vi "界面设计_灯.vi"(11 "停止":bool) -> (0 "布尔":bool, 1 "布尔 2":bool, 2 "布尔 4":bool, 3 "布尔 3":bool, 6 "布尔 5":bool, 8 "布尔 6":bool, 10 "布尔 8":bool, 12 "布尔 7":bool, 14 "布尔 9":bool, 15 "布尔 10":bool, 16 "布尔 12":bool, 17 "布尔 11":bool)   [LabVIEW 2019]
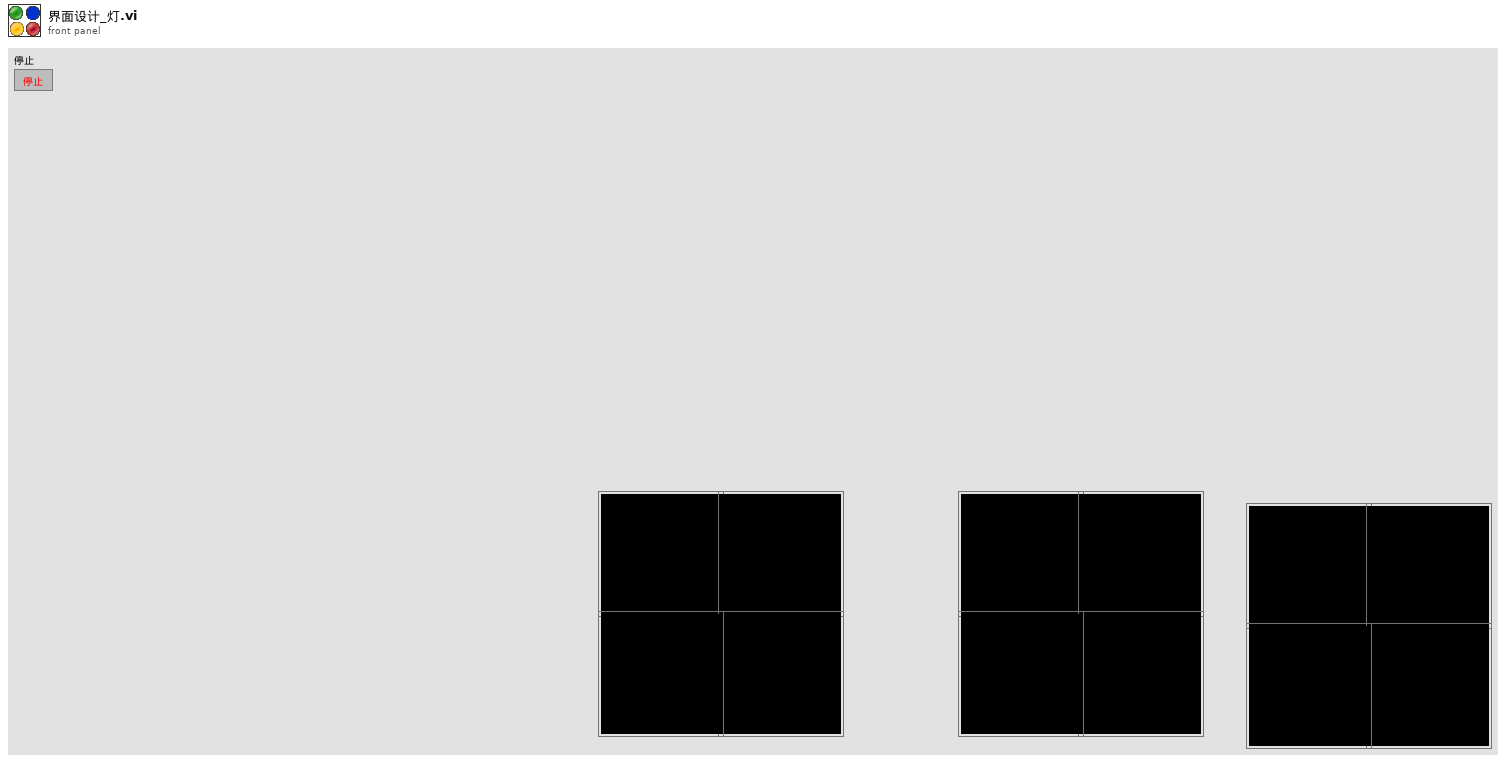
[diagram p1: front panel]
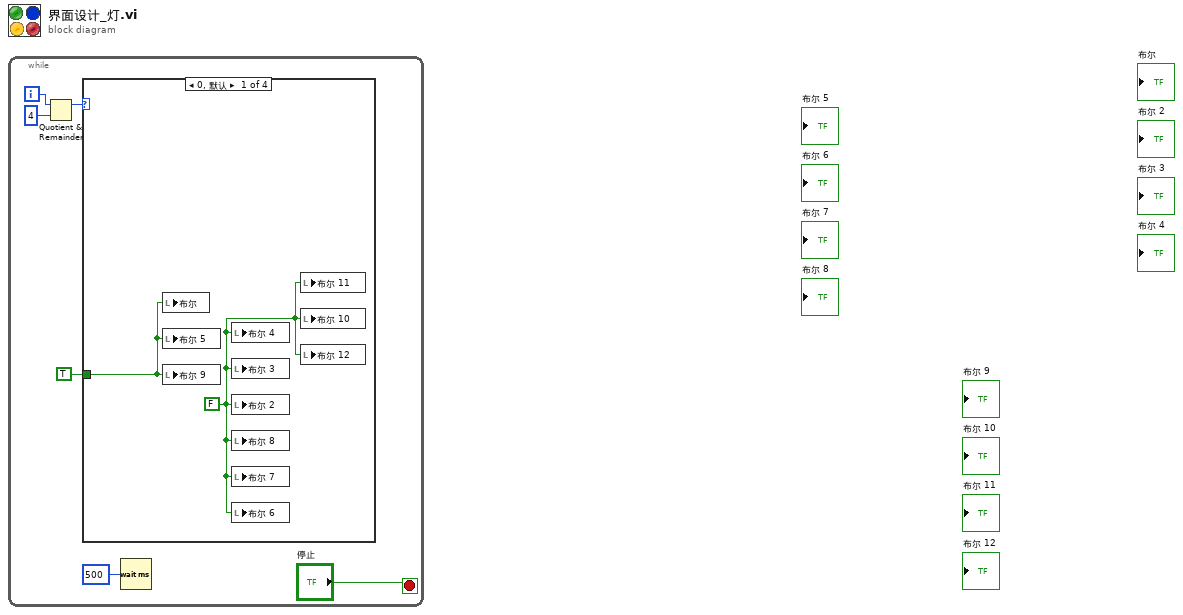
[diagram p0: block diagram]
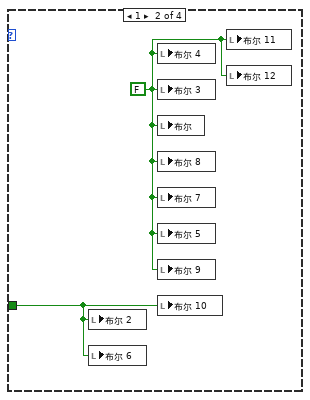
[diagram p2: hidden frame]
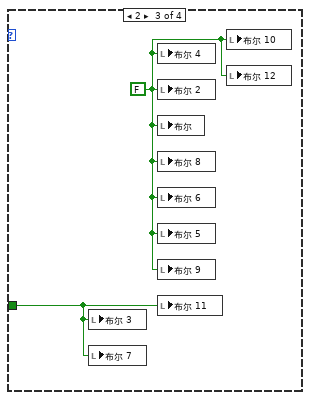
[diagram p3: hidden frame]
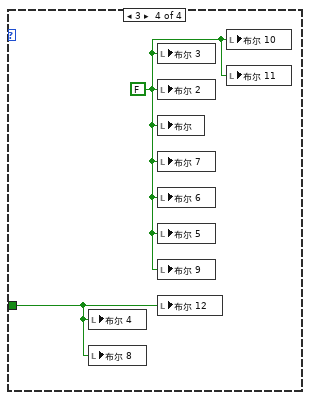
[diagram p4: hidden frame]
diagram:
  n1 = while {
    i -> [w5]
    stop <- "停止" stop-if-true
    n2 = Quotient & Remainder(x=w5, y=4) -> (x-y*floor(x/y)=w3:i32)  [unwired: 1 out]
    n3 = case shown="0, 默认" w3 {
      tunnel: TRUE ("布尔 4") -> [w8 w10 w12 w14]
      frame 0, Default {
        w7 = FALSE ("布尔 2")
        n4 = local write "布尔"(w8) -> ()
        n5 = local write "布尔 5"(w8) -> ()
        n6 = local write "布尔 9"(w8) -> ()
        n7 = local write "布尔 4"(w7) -> ()
        n8 = local write "布尔 3"(w7) -> ()
        n9 = local write "布尔 2"(w7) -> ()
        n10 = local write "布尔 8"(w7) -> ()
        n11 = local write "布尔 7"(w7) -> ()
        n12 = local write "布尔 6"(w7) -> ()
        n13 = local write "布尔 11"(w7) -> ()
        n14 = local write "布尔 10"(w7) -> ()
        n15 = local write "布尔 12"(w7) -> ()
      }
      frame 1 {
        w9 = FALSE ("布尔")
        n16 = local write "布尔 2"(w10) -> ()
        n17 = local write "布尔 6"(w10) -> ()
        n18 = local write "布尔 4"(w9) -> ()
        n19 = local write "布尔 3"(w9) -> ()
        n20 = local write "布尔"(w9) -> ()
        n21 = local write "布尔 8"(w9) -> ()
        n22 = local write "布尔 7"(w9) -> ()
        n23 = local write "布尔 5"(w9) -> ()
        n24 = local write "布尔 9"(w9) -> ()
        n25 = local write "布尔 10"(w10) -> ()
        n26 = local write "布尔 11"(w9) -> ()
        n27 = local write "布尔 12"(w9) -> ()
      }
      frame 2 {
        w11 = FALSE ("布尔 4")
        n28 = local write "布尔 3"(w12) -> ()
        n29 = local write "布尔 7"(w12) -> ()
        n30 = local write "布尔 4"(w11) -> ()
        n31 = local write "布尔 2"(w11) -> ()
        n32 = local write "布尔"(w11) -> ()
        n33 = local write "布尔 8"(w11) -> ()
        n34 = local write "布尔 6"(w11) -> ()
        n35 = local write "布尔 5"(w11) -> ()
        n36 = local write "布尔 9"(w11) -> ()
        n37 = local write "布尔 11"(w12) -> ()
        n38 = local write "布尔 10"(w11) -> ()
        n39 = local write "布尔 12"(w11) -> ()
      }
      frame 3 {
        w13 = FALSE ("布尔 3")
        n40 = local write "布尔 4"(w14) -> ()
        n41 = local write "布尔 8"(w14) -> ()
        n42 = local write "布尔 3"(w13) -> ()
        n43 = local write "布尔 2"(w13) -> ()
        n44 = local write "布尔"(w13) -> ()
        n45 = local write "布尔 7"(w13) -> ()
        n46 = local write "布尔 6"(w13) -> ()
        n47 = local write "布尔 5"(w13) -> ()
        n48 = local write "布尔 9"(w13) -> ()
        n49 = local write "布尔 12"(w14) -> ()
        n50 = local write "布尔 10"(w13) -> ()
        n51 = local write "布尔 11"(w13) -> ()
      }
    }
    n52 = Wait (ms)(milliseconds to wait=u32 500 ("等待时间（毫秒）")) -> ()  [unwired: 1 out]
  }
